vi "Is Same Object.vi"(8 "error in (no error)":errorcluster, 10 "values":refnum<vi>, 11 "GObject in":refnum<vi>) -> (0 "error out":errorcluster, 2 "Same":bool)   [LabVIEW 2025, in "Scripting Server.lvlib"]
uses:
  Scripting Server.lvlib
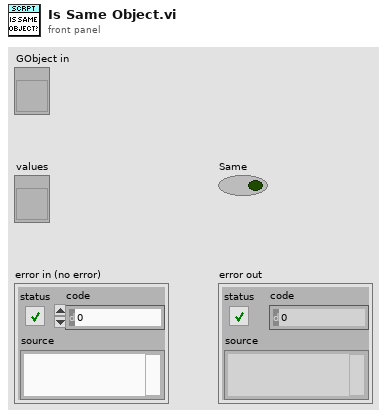
[diagram p1: front panel]
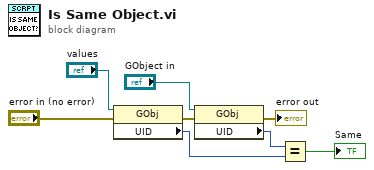
[diagram p0: block diagram]
diagram:
  n1 = property class="GObj"(reference="values", error in="error in (no error)") -> (error out=w6:errorcluster, "UID"=w8:i32)  [unwired: 1 out]
  n2 = property class="GObj"(reference="GObject in", error in=w6) -> (error out=→"error out":errorcluster, "UID"=w4:i32)  [unwired: 1 out]
  n3 = Equal?(x=w4, y=w8) -> (x = y?=→"Same":bool)
